vi "usrp_mimo_ofdm_2x1.vi"() -> ()   [LabVIEW 2014]
uses:
  <instrlib>/niUSRP/niUSRP Timestamp.ctl
  <vilib>/addons/Modulation/Analog/controls/Complex Data Waveform.ctl
  <vilib>/addons/Modulation/Digital/General/MT Generate Bits (Galois, PN Order).vi
  <vilib>/addons/Modulation/Digital/Support/Common/Validators/mod_Generate Bits Validate.vi
  <vilib>/addons/Modulation/Analog/support/mod_Set Error Source.vi
  <instrlib>/niUSRP/niUSRP Configure Time Start Trigger.vi
  <vilib>/addons/Modulation/Digital/General/MT Generate QAM System Parameters(M).vi
  <vilib>/addons/Modulation/Digital/Support/Common/Validators/mod_Generate Filter Coefficients Validate.vi
  <vilib>/addons/Modulation/Digital/General/subVIs/mod_Generate Filter Coefficients.vi
  <vilib>/addons/Modulation/Digital/General/subVIs/mod_Generate Bits PN Sequence.vi
  <vilib>/addons/Modulation/Digital/General/MT Map Bits to QAM Symbols.vi
  <vilib>/addons/Modulation/Digital/General/MT Apply Pulse Shaping Filter (Generic).vi
  <instrlib>/niUSRP/niUSRP Write Tx Data (2D CDB).vi
  <instrlib>/niUSRP/niUSRP Fetch Rx Data (2D CDB).vi
  <vilib>/addons/Modulation/Digital/General/MT Apply Matched Filter (Generic).vi
  <vilib>/addons/Modulation/Digital/General/MT Align to Ideal Symbols (Generic).vi
  <vilib>/measure/maspectr.llb/FFT Power Spectrum and PSD for 1 Chan (CDB).vi
  <vilib>/addons/Modulation/Digital/General/MT Map QAM Symbols to Bits.vi
  <vilib>/addons/Modulation/niDMT.lvlib
  <vilib>/measure/NI_MAPro.lvlib
  <vilib>/addons/Modulation/niAMT.lvlib
panel:
  out "Waveform Chart":i16(graph)
  out "size(s) 2":i32
  out "size(s) 3":i32[](array[numeric])
  out "sum":i16
  out "size(s)":i32
  out "x = 0?":bool
  out "input bits stream":i8[](array[numeric]) caption="input bit stream"
  out "output bit stream":i8[](array[numeric])
  in  "CP length":u32=32 caption="CP Size"
  in  "Message Carrier":u32=128
  in  "FFT Size":u32=256
  in  "RXa:Timebase Clock Source":string(combo)="Internal"
  in  "RXa:Reference Frequency Source":string(combo)="Internal"
  in  "TXa:Timebase Clock Source":string(combo)="Internal"
  in  "TXa:Reference Frequency Source":string(combo)="Internal"
  out "OFF":bool=TRUE
  out "RX error":bool
  out "TX error":bool
  out "ERROR":bool
  out "Decoded Constellation Map":cdb[](graph)
  in  "TX timeout":dbl=10.0
  out "error IO":errorcluster
  in  "stop":bool
  out "Transmitted Constellation Map":cluster{dbl[], dbl[]}[](graph)
  out "PSD of Received Signal":cluster{"f0":dbl, "df":dbl, "magnitude":dbl[]}[](graph)
  out "USRP timestamp":T1={"whole seconds"=11, "fractional seconds"=0.9000012199999999}
  in  "number of samples":i64=100000
  in  "M-QAM (16)":i32=16
  in  "total bits (128)":i32=512 caption="total bits (512)"
  in  "filter length (symbols)":i32=8
  in  "filter parameter":dbl=0.5 format="%.2f"
  in  "samples per symbol (16)":i32=4
  in  "pulse shaping filter (none)":T2(ring)=enum."Raised Cosine"
  in  "RXb:Timebase Clock Source":string(combo)="Mimo"
  in  "RXb:Reference Frequency Source":string(combo)="Mimo"
  in  "TXb:Timebase Clock Source":string(combo)="Mimo"
  in  "TXb:Reference Frequency Source":string(combo)="Mimo"
  in  "RXb Active Antenna":string="RX2"
  in  "TXb Active Antenna":string="TX1"
  in  "RXb Gain":dbl
  in  "TXb Gain":dbl
  in  "RXa Active Antenna":string="RX2"
  in  "RXa Gain":dbl
  in  "TXa Active Antenna":string="TX1"
  in  "TXa Gain":dbl
  in  "Carrier Frequency":dbl=1200000000.0 format="%#_6p"
  in  "IQ Rate":dbl=1000000.0 format="%#_6p"
  in  "TX device names":refnum<k15>="192.168.10.2;192.168.10.5"
  in  "start trigger time":T1={"whole seconds"=4, "fractional seconds"=0.1}
  in  "RX device names":refnum<k15>="192.168.10.2;192.168.10.5"
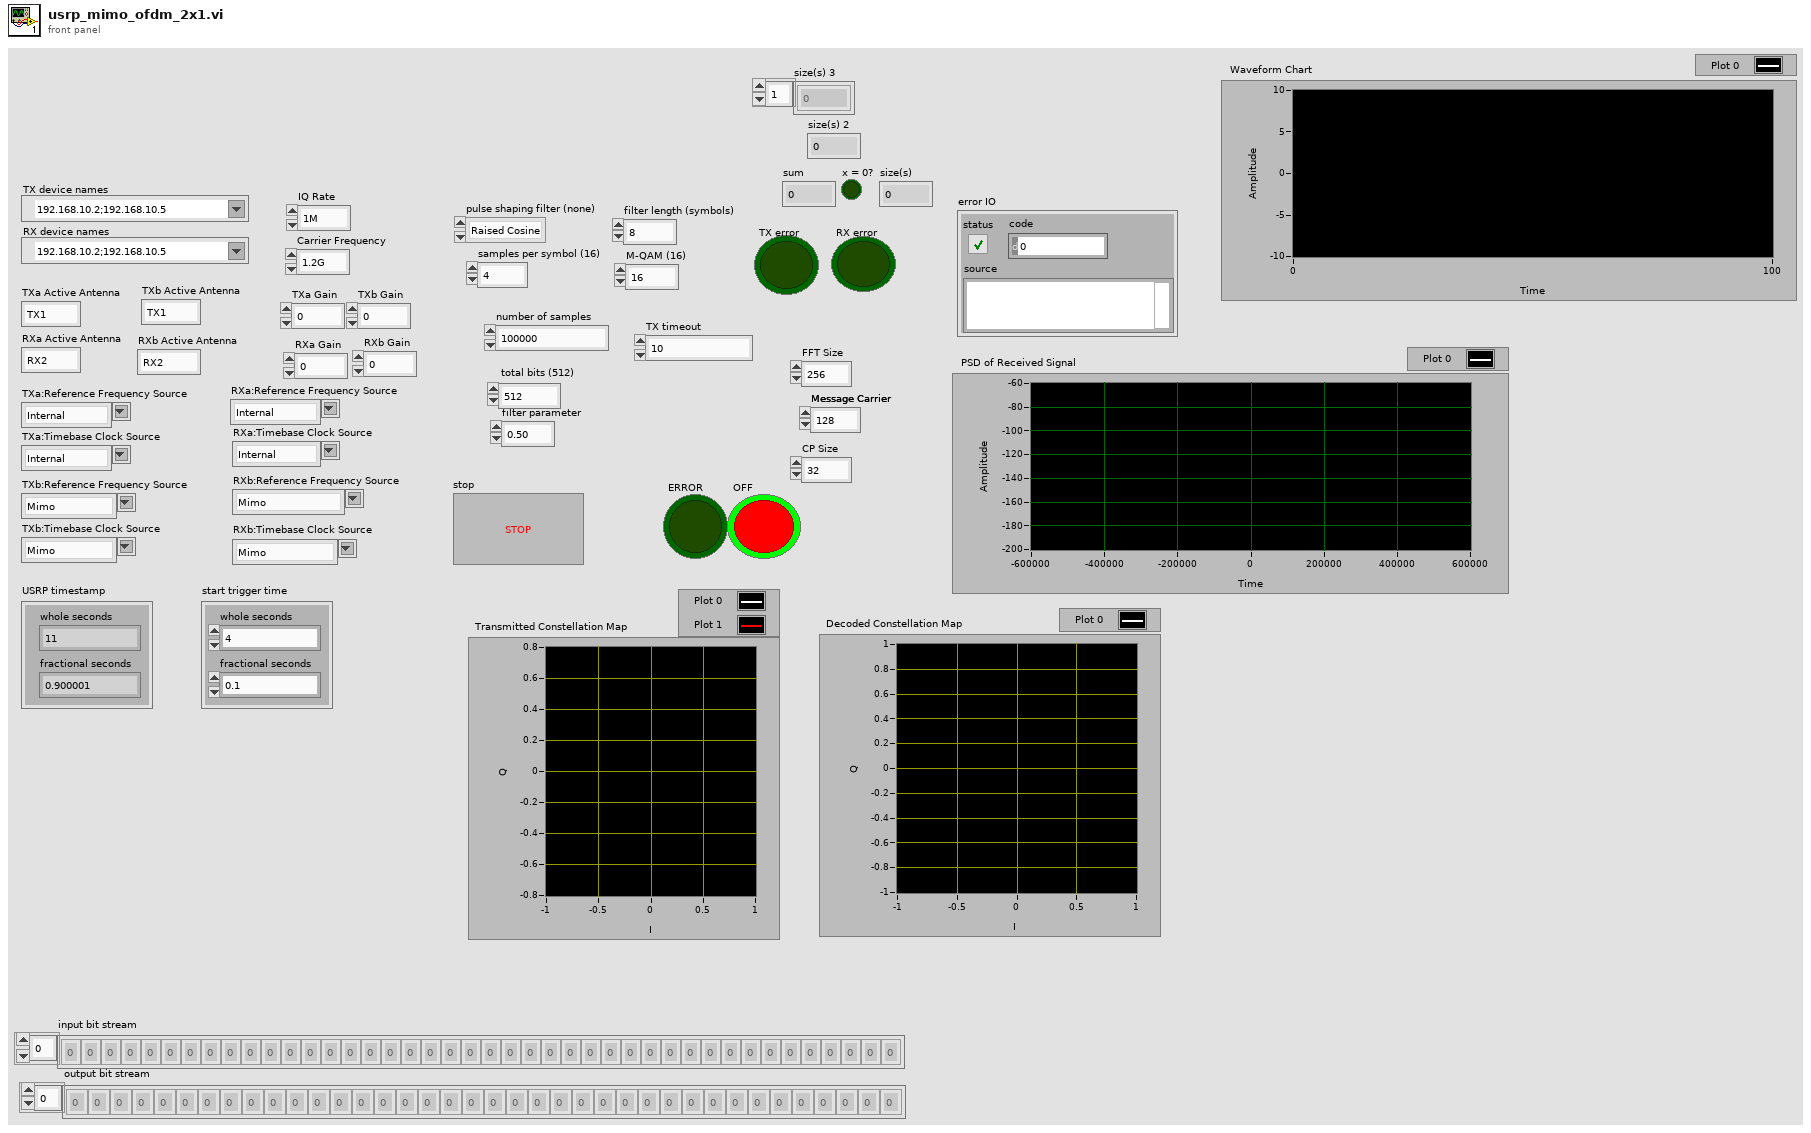
[diagram p1: front panel]
types:
  T1 = typedef "niUSRP Timestamp.ctl" = cluster{"whole seconds":u64, "fractional seconds":dbl}
  T2 = enum16{"none", "Raised Cosine", "Root Raised Cos", "Gaussian"}
  T3 = enum16{"FSK", "PSK", "QAM", "MSK", "PAM", "ASK", "CPM"}
  T4 = cluster{"samples per symbol (16)":i32, "symbol map":cdb[]}
  T5 = typedef "niAMT.lvlib/Complex Data Waveform.ctl" = cluster{"t0":dbl, "dt":dbl, "Y":cdb[]}
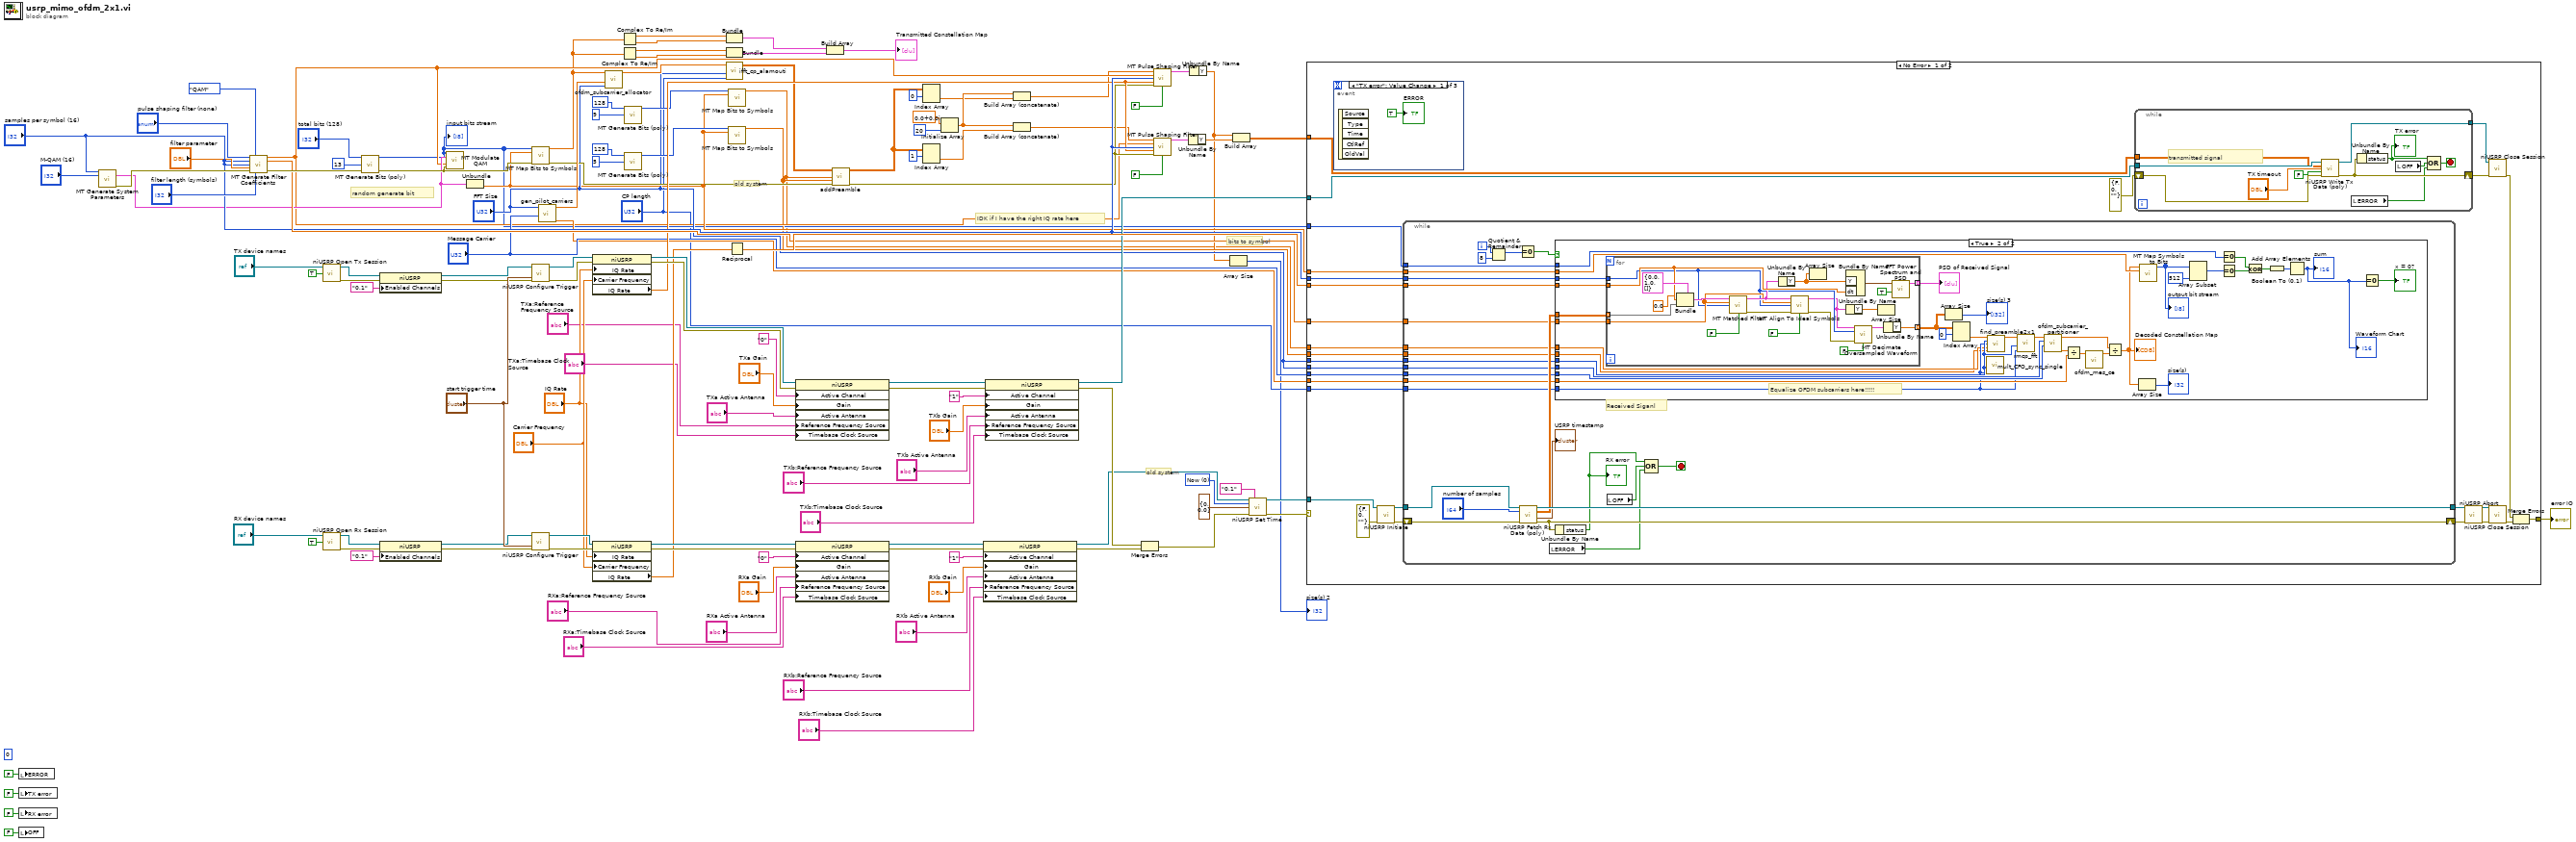
[diagram p0: block diagram]
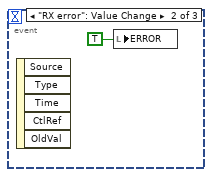
[diagram p2: hidden frame]
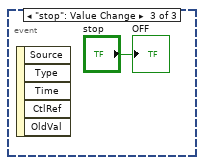
[diagram p3: hidden frame]
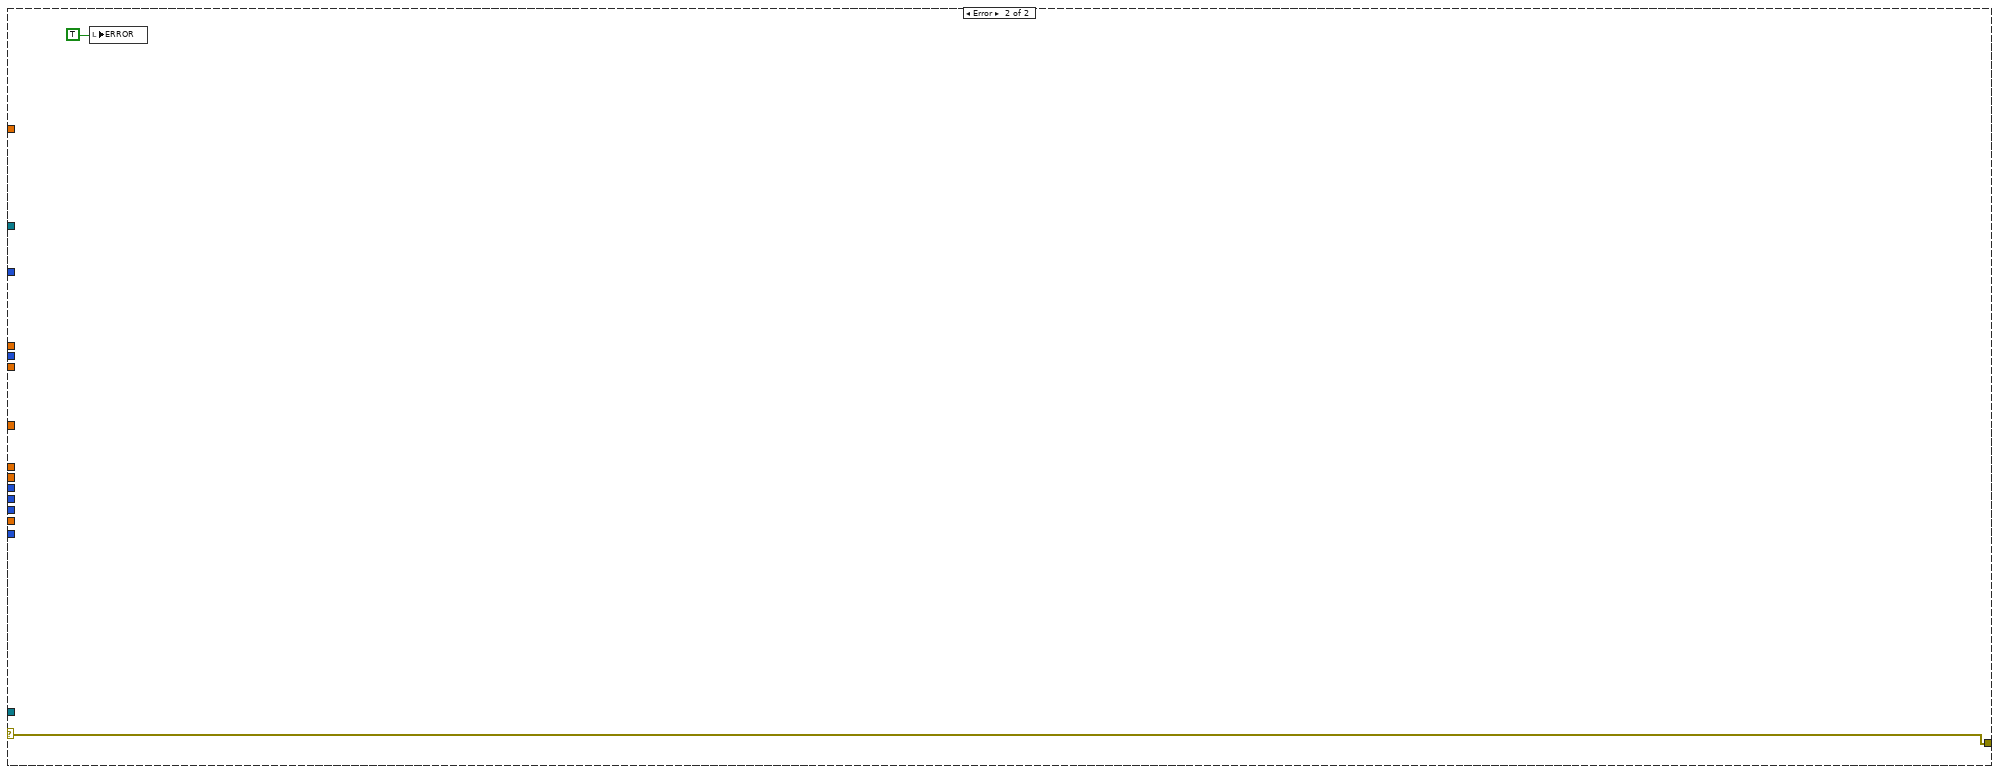
[diagram p5: hidden frame]
diagram:
  (unwired) 0 ("index")
  w85 = 0 items=["Now", "Next Timebase Edge"] ("apply timestamp")
  # "IDK if I have the right IQ rate here"
  # "bits to symbol"
  # "old system"
  # "old system"
  # "random generate bit"
  n1 = local write "ERROR"(FALSE) -> ()
  n2 = local write "TX error"(FALSE) -> ()
  n3 = local write "RX error"(FALSE) -> ()
  n4 = local write "OFF"(FALSE) -> ()
  n5 = call-poly <vilib>:"MT Generate System Parameters.vi"("samples per symbol (16)"="samples per symbol (16)", "M-QAM (16)"="M-QAM (16)") -> ("QAM system parameters"=w27:T4, "error out"=w75:errorcluster)  [unwired: 11 in, 1 out]
  n6 = call <vilib>:"MT Generate Filter Coefficients.vi"("pulse shaping filter (none)"="pulse shaping filter (none)", "modulation type"=T3."QAM", "pulse shaping samples per symbol (16)"="samples per symbol (16)", "matched samples per symbol (16)"="samples per symbol (16)", "filter parameter"="filter parameter", "error in (no error)"=w75, "filter length (symbols)"="filter length (symbols)") -> ("pulse shaping filter coefficients"=w18:dbl[], "matched filter coefficients"=w53:dbl[], "error out"=w74:errorcluster)  [unwired: 6 in]
  n7 = call <instrlib>:"niUSRP Open Tx Session.vi"("device names"="TX device names", "reset"=TRUE) -> ("session handle out"=w58:refnum<k15>, "error out"=w57:errorcluster)  [unwired: 12 in]
  n8 = call <instrlib>:"niUSRP Open Rx Session.vi"("device names"="RX device names", "reset"=TRUE) -> ("session handle out"=w60:refnum<k15>, "error out"=w59:errorcluster)  [unwired: 12 in]
  n9 = call-poly <vilib>:"MT Generate Bits (poly).vi"("total bits (128)"="total bits (128)", "PN sequence order (9)"=13, "error in (no error)"=w74) -> ("output bit stream"=w15:i8[], "error out"=w44:errorcluster)  [unwired: 10 in, 1 out]
  "input bits stream" <- w15
  n10 = property class="niUSRP"(reference=w58, error in=w57, "Enabled Channels"="0,1" ("Configuration:Enabled Channels")) -> (reference out=w119:refnum<k15>, error out=w118:errorcluster)
  n11 = property class="niUSRP"(reference=w60, error in=w59, "Enabled Channels"="0,1" ("Configuration:Enabled Channels")) -> (reference out=w117:refnum<k15>, error out=w116:errorcluster)
  n12 = call <vilib>:"MT Modulate QAM.vi"("input bit stream"=w15, "QAM system parameters"=w27, "pulse shaping filter coefficients"=w18, "error in (no error)"=w44) -> ()  [unwired: 9 in, 3 out]
  n13 = Unbundle(w27) -> ("symbol map"=w21:cdb[])  [unwired: 1 out]
  n14 = call-poly <instrlib>:"niUSRP Configure Trigger.vi"("session handle"=w119, "start trigger time"="start trigger time", "error in (no error)"=w118) -> ("session handle out"=w111:refnum<k15>, "error out"=w110:errorcluster)  [unwired: 11 in]
  n15 = call-poly <instrlib>:"niUSRP Configure Trigger.vi"("session handle"=w117, "start trigger time"="start trigger time", "error in (no error)"=w116) -> ("session handle out"=w115:refnum<k15>, "error out"=w114:errorcluster)  [unwired: 11 in]
  n16 = call-poly <vilib>:"MT Map Bits to Symbols.vi"("input bit stream"=w15, "symbol map"=w21, "error in (no error)"=w44) -> ("symbols"=w16:cdb[], "error out"=w31:errorcluster)  [unwired: 11 in]
  n17 = call "gen_pilot_carriers.vi"("message carrier"="Message Carrier", "FFT size"="FFT Size") -> ("RX pilot carriers"=w22:cdb[], "TX pilot carriers"=w43:cdb[])  [unwired: 8 in]
  n18 = property class="niUSRP"(reference=w111, error in=w110, "IQ Rate"="IQ Rate", "Carrier Frequency"="Carrier Frequency") -> (reference out=w107:refnum<k15>, error out=w106:errorcluster, "IQ Rate"=w38:dbl)
  n19 = property class="niUSRP"(reference=w115, error in=w114, "IQ Rate"="IQ Rate", "Carrier Frequency"="Carrier Frequency") -> (reference out=w113:refnum<k15>, error out=w112:errorcluster, "IQ Rate"=w70:dbl)
  n20 = call "ofdm_subcarrier_allocator.vi"("fft size"="FFT Size", "pilot symbol"=w43, "message symbol"=w16) -> ("OFDM symbol"=w42:cdb[])  [unwired: 8 in]
  n21 = Complex To Re/Im(x + iy=w16) -> (x=w68:dbl[], y=w67:dbl[])
  n22 = Complex To Re/Im(x + iy=w16) -> (x=w66:dbl[], y=w65:dbl[])
  n23 = call-poly <vilib>:"MT Generate Bits (poly).vi"("total bits (128)"=128, "PN sequence order (9)"=9) -> ("output bit stream"=w24:i8[])  [unwired: 11 in, 2 out]
  n24 = call-poly <vilib>:"MT Generate Bits (poly).vi"("total bits (128)"=128, "PN sequence order (9)"=5) -> ("output bit stream"=w26:i8[])  [unwired: 11 in, 2 out]
  n25 = Bundle(w68, w67) -> (w63:cluster{dbl[], dbl[]})  [unwired: 1 in]
  n26 = Bundle(w66, w65) -> (w64:cluster{dbl[], dbl[]})  [unwired: 1 in]
  n27 = call "ifft_cp_alamouti.vi"("CP Length"="CP length", "FFT Size"="FFT Size", "Modulated Stream"=w42) -> ("Baseband Streams"=w33:cdb[][])  [unwired: 8 in]
  n28 = call-poly <vilib>:"MT Map Bits to Symbols.vi"("input bit stream"=w24, "symbol map"=w21) -> ("symbols"=w1:cdb[])  [unwired: 12 in, 1 out]
  n29 = call-poly <vilib>:"MT Map Bits to Symbols.vi"("input bit stream"=w26, "symbol map"=w21) -> ("symbols"=w17:cdb[])  [unwired: 12 in, 1 out]
  n30 = Reciprocal(x=w70) -> (1/x=w69:dbl)
  n31 = property class="niUSRP"(reference=w107, error in=w106, "Active Channel"="0", "Gain"="TXa Gain", "Active Antenna"="TXa Active Antenna", "Reference Frequency Source"="TXa:Reference Frequency Source", "Timebase Clock Source"="TXa:Timebase Clock Source") -> (reference out=w97:refnum<k15>, error out=w96:errorcluster)
  n32 = property class="niUSRP"(reference=w113, error in=w112, "Active Channel"="0", "Gain"="RXa Gain", "Active Antenna"="RXa Active Antenna", "Reference Frequency Source"="RXa:Reference Frequency Source", "Timebase Clock Source"="RXa:Timebase Clock Source") -> (reference out=w99:refnum<k15>, error out=w98:errorcluster)
  n33 = Build Array(w63, w64) -> (→"Transmitted Constellation Map":cluster{dbl[], dbl[]}[])
  n34 = call "addPreamble.vi"("Input Symbol Stream"=w33, "Training Sequence"=w1, "Training Sequence 2"=w17, "error in (no error)"=w31) -> ("Output Transmit \nPackets"=w32:cdb[][], "error out"=w30:errorcluster)  [unwired: 10 in]
  n35 = Index Array(array=w32, index (row)=0) -> (element=w2:cdb[])  [unwired: 1 in]
  n36 = Index Array(array=w32, index (row)=1) -> (element=w3:cdb[])  [unwired: 1 in]
  n37 = Initialize Array(cdb 0.0+0.0i ("element"), 20 ("dimension size")) -> (w4:cdb[])
  n38 = property class="niUSRP"(reference=w99, error in=w98, "Active Channel"="1", "Gain"="RXb Gain", "Active Antenna"="RXb Active Antenna", "Reference Frequency Source"="RXb:Reference Frequency Source", "Timebase Clock Source"="RXb:Timebase Clock Source") -> (reference out=w55:refnum<k15>, error out=w83:errorcluster)
  n39 = property class="niUSRP"(reference=w97, error in=w96, "Active Channel"="1", "Gain"="TXb Gain", "Active Antenna"="TXb Active Antenna", "Reference Frequency Source"="TXb:Reference Frequency Source", "Timebase Clock Source"="TXb:Timebase Clock Source") -> (reference out=w56:refnum<k15>, error out=w82:errorcluster)
  n40 = Build Array (concatenate)(w4, w2) -> (w6:cdb[])
  n41 = Build Array (concatenate)(w4, w3) -> (w5:cdb[])
  n42 = Merge Errors(w82, w83) -> (w81:errorcluster)
  n43 = call-poly <vilib>:"MT Pulse Shaping Filter.vi"("symbols"=w6, "pulse shaping filter coefficients"=w18, "samples per symbol (16)"="samples per symbol (16)", "symbol rate (Hz)"=w38, "error in (no error)"=w30, "reset? (T)"=FALSE) -> ("output complex waveform"=w36:T5)  [unwired: 8 in, 1 out]
  n44 = call-poly <vilib>:"MT Pulse Shaping Filter.vi"("symbols"=w5, "pulse shaping filter coefficients"=w18, "samples per symbol (16)"="samples per symbol (16)", "symbol rate (Hz)"=w38, "error in (no error)"=w30, "reset? (T)"=FALSE) -> ("output complex waveform"=w35:T5)  [unwired: 8 in, 1 out]
  n45 = Unbundle By Name(w35) -> ("Y"=w34:cdb[])
  n46 = Unbundle By Name(w36) -> ("Y"=w10:cdb[])
  n47 = Array Size(array=w10) -> (size(s)=→"size(s) 2":i32)
  n48 = Build Array(w10, w34) -> (w13:cdb[][])
  n49 = call <instrlib>:"niUSRP Set Time.vi"("session handle"=w55, "channel list"="0,1" ("Configuration:Enabled Channels"), "apply timestamp"=w85, "timestamp"=T1 {"whole seconds"=0, "fractional seconds"=0.0}, "error in (no error)"=w81) -> ("session handle out"=w54:refnum<k15>, "error out"=w80:errorcluster)  [unwired: 9 in]
  n50 = case shown="No Error" w80 {
    selector: w80 -> [_ w253]
    tunnel: w54 -> [w140 _]
    tunnel: w56 -> [w153 _]
    tunnel: w13 -> [w154 _]
    tunnel: w69 -> [w144 _]
    tunnel: [w141 w253] -> w62
    tunnel: w53 -> [w137 _]
    tunnel: "samples per symbol (16)" -> [w136 _]
    tunnel: "FFT Size" -> [w135 _]
    tunnel: "Message Carrier" -> [w134 _]
    tunnel: w1 -> [w133 _]
    tunnel: w17 -> [w132 _]
    tunnel: "FFT Size" -> [w131 _]
    tunnel: "CP length" -> [w130 _]
    tunnel: w22 -> [w129 _]
    tunnel: w21 -> [w128 _]
    tunnel: w15 -> [w127 _]
    frame No Error {
      n51 = event shown="[0] \"TX error\": Value Change" {
        selector: _ -> [_ _ _]
        dyn-events: _ -> [_ _ _]
        timeout: _ -> [_ _ _]
        event "TX error": Value Change {
          n52 = event-data() -> ()  [unwired: 1 in, 5 out]
          "ERROR" <- TRUE
        }
        event "RX error": Value Change {
          n53 = event-data() -> ()  [unwired: 1 in, 5 out]
          n54 = local write "ERROR"(TRUE) -> ()
        }
        event "stop": Value Change {
          n55 = event-data() -> ()  [unwired: 1 in, 5 out]
          "OFF" <- "stop"
        }
      }
      n56 = call <instrlib>:"niUSRP Initiate.vi"("session handle"=w140, "error in (no error)"=errorcluster {"status"=FALSE, "code"=0, "source"=""}) -> ("session handle out"=w152:refnum<k15>, "error out"=w151:errorcluster)  [unwired: 12 in]
      n57 = while {
        tunnel: w152 -> [w183]
        shift-right: [w177] -> w150
        shift-left: w151 -> [w182]
        tunnel: [w181] -> w149
        tunnel: w144 -> [w178]
        tunnel: w137 -> [w174]
        tunnel: w136 -> [w173]
        tunnel: w135 -> [w170]
        tunnel: w134 -> [w169]
        tunnel: w133 -> [w168]
        tunnel: w132 -> [w167]
        tunnel: w131 -> [w166]
        tunnel: w130 -> [w165]
        tunnel: w129 -> [w164]
        tunnel: w128 -> [w163]
        tunnel: w127 -> [w162]
        i -> [w161]
        stop <- w175 stop-if-true
        # "Received Siganl"
        n58 = Quotient & Remainder(x=w161, y=8) -> (x-y*floor(x/y)=w159:i32)  [unwired: 1 out]
        n59 = Equal To 0?(x=w159) -> (x = 0?=w158:bool)
        n60 = call-poly <instrlib>:"niUSRP Fetch Rx Data (poly).vi"("session handle"=w183, "number of samples"="number of samples", "error in (no error)"=w182) -> ("session handle out"=w181:refnum<k15>, "data"=w179:cdb[][], "timestamp"=→"USRP timestamp":T1, "error out"=w177:errorcluster)  [unwired: 9 in]
        n61 = local read "ERROR"() -> (w172:bool)
        n62 = case shown="True" w158 {
          tunnel: w179 -> [_ w217]
          tunnel: w178 -> [_ w219]
          tunnel: w174 -> [_ w216]
          tunnel: w173 -> [_ w215]
          tunnel: w170 -> [_ w214]
          tunnel: w169 -> [_ w213]
          tunnel: w168 -> [_ w188]
          tunnel: w167 -> [_ w187]
          tunnel: w166 -> [_ w190]
          tunnel: w165 -> [_ w189]
          tunnel: w164 -> [_ w212]
          tunnel: w163 -> [_ w211]
          tunnel: w162 -> [_ w200]
          frame False {
          }
          frame True {
            # "Equalize OFDM subcarriers here!!!!!"
            n63 = for {
              tunnel: w219 -> [w236]
              tunnel: [w238] -> w218 mode=indexing
              tunnel: w217 -> [w235] mode=indexing
              tunnel: w216 -> [w231]
              tunnel: w215 -> [w228]
              tunnel: [w220] -> w193 mode=indexing
              n64 = Bundle(cluster=T5 {"t0"=0.0, "dt"=1.0, "Y"=[]} ("input complex waveform"), "t0"=0.0, "dt"=w236, "Y"=w235) -> (w233:T5)
              n65 = call-poly <vilib>:"MT Matched Filter.vi"("input complex waveform"=w233, "matched filter coefficients"=w231, "samples per symbol (16)"=w228, "reset? (T)"=FALSE) -> ("output complex waveform"=w232:T5, "error out"=w230:errorcluster)  [unwired: 10 in]
              n66 = Unbundle By Name(w232) -> ("Y"=w223:cdb[])
              n67 = call-poly <vilib>:"MT Align To Ideal Symbols.vi"("input complex waveform"=w232, "matched filter coefficients"=w231, "samples per symbol (16)"=w228, "error in (no error)"=w230, "reset? (T)"=FALSE) -> ("output complex waveform"=w222:T5, "error out"=w229:errorcluster)  [unwired: 8 in, 1 out]
              n68 = Array Size(array=w223) -> ()  [unwired: 1 out]
              n69 = Bundle By Name("Y"=w223, "dt"=w236) -> (w240:waveform(cdb))  [unwired: 1 in]
              n70 = Unbundle By Name(w222) -> ("Y"=w221:cdb[])
              n71 = call <vilib>:"MT Decimate Oversampled Waveform.vi"("input complex waveform"=w222, "decimation factor"=w228, "error in (no error)"=w229, "reset? (T)"=FALSE) -> ("output complex waveform"=w227:T5)  [unwired: 10 in, 1 out]
              n72 = Array Size(array=w221) -> ()  [unwired: 1 out]
              n73 = Unbundle By Name(w227) -> ("Y"=w220:cdb[])
              n74 = call-poly <vilib>:"FFT Power Spectrum and PSD.vi"("dB On (F)"=TRUE, "time signal"=w240) -> ("Power Spectrum / PSD"=w238:cluster{"f0":dbl, "df":dbl, "magnitude":dbl[]})  [unwired: 6 in, 3 out]
            }
            "PSD of Received Signal" <- w218
            n75 = Array Size(array=w193) -> (size(s)=→"size(s) 3":i32[])
            n76 = Index Array(array=w193, index (row)=0) -> (element=w191:cdb[])  [unwired: 1 in]
            n77 = call "mult_CFO_sync_single.vi"("CP length"=w189, "FFT size"=w190) -> ()  [unwired: 9 in, 1 out]
            n78 = call "find_preamble2x1.vi"("received \ntime symbol"=w191, "FFT Size"=w190, "CP Length"=w189, "1st preamble"=w188, "2nd preamble"=w187) -> ("OFDM Symbol"=w186:cdb[])  [unwired: 10 in]
            n79 = call "rmcp_fft.vi"("CP length"=w189, "fft size"=w190, "time symbol"=w186) -> ("freq output"=w202:cdb[])  [unwired: 8 in]
            n80 = call "ofdm_subcarrier_partitioner.vi"("message carrier"=w213, "FFT size"=w214, "received symbol"=w202) -> ("pilot subcarriers"=w207:cdb[], "message subcarriers"=w204:cdb[])  [unwired: 7 in]
            n81 = Divide(x=w207, y=w212) -> (x/y=w206:cdb[])
            n82 = call "ofdm_mes_ce.vi"("ZF \nchannel \nestimates"=w206) -> ("interpolated\n mes carrier CE"=w205:cdb[])  [unwired: 10 in]
            n83 = Divide(x=w204, y=w205) -> (x/y=w201:cdb[])
            "Decoded Constellation Map" <- w201
            n84 = Array Size(array=w201) -> (size(s)=→"size(s)":i32)
            n85 = call-poly <vilib>:"MT Map Symbols to Bits.vi"("symbols"=w201, "symbol map"=w211) -> ("output bit stream"=w209:i8[])  [unwired: 12 in, 1 out]
            "output bit stream" <- w209
            n86 = Array Subset(array=w209, length=512) -> (w198:i8[])  [unwired: 1 in]
            n87 = Equal To 0?(x=w200) -> (x = 0?=w197:bool[])
            n88 = Equal To 0?(x=w198) -> (x = 0?=w199:bool[])
            n89 = Exclusive Or(1:w199, 2:w197) -> (0:w196:bool[])
            n90 = Boolean To (0,1)(Boolean=w196) -> (0, 1=w195:i16[])
            n91 = Add Array Elements(numeric array=w195) -> (sum=w185:i16)
            "sum" <- w185
            "Waveform Chart" <- w185
            n92 = Equal To 0?(x=w185) -> (x = 0?=→"x = 0?":bool)
          }
        }
        n93 = Unbundle By Name(w177) -> ("status"=w176:bool)
        "RX error" <- w176
        n94 = local read "OFF"() -> (w171:bool)
        n95 = Compound Arithmetic op=OR(w176, w171, w172) -> (w175:bool)
      }
      n96 = while {
        tunnel: w154 -> [w247]
        tunnel: w153 -> [w251]
        tunnel: [w250] -> w146
        shift-right: [w246] -> w145
        shift-left: errorcluster {"status"=FALSE, "code"=0, "source"=""} ("error out") -> [w249]
        stop <- w244 stop-if-true
        # "transmitted signal"
        n97 = call-poly <instrlib>:"niUSRP Write Tx Data (poly).vi"("session handle"=w251, "data"=w247, "timeout"="TX timeout", "end of data?"=FALSE, "error in (no error)"=w249) -> ("session handle out"=w250:refnum<k15>, "error out"=w246:errorcluster)  [unwired: 9 in]
        n98 = local read "ERROR"() -> (w242:bool)
        n99 = Unbundle By Name(w246) -> ("status"=w245:bool)
        "TX error" <- w245
        n100 = local read "OFF"() -> (w241:bool)
        n101 = Compound Arithmetic op=OR(w245, w241, w242) -> (w244:bool)
      }
      n102 = call <instrlib>:"niUSRP Abort.vi"("session handle"=w149, "error in (no error)"=w150) -> ("session handle out"=w148:refnum<k15>, "error out"=w147:errorcluster)  [unwired: 12 in]
      n103 = call <instrlib>:"niUSRP Close Session.vi"("session handle"=w146, "error in (no error)"=w145) -> ("error out"=w142:errorcluster)  [unwired: 13 in]
      n104 = call <instrlib>:"niUSRP Close Session.vi"("session handle"=w148, "error in (no error)"=w147) -> ("error out"=w143:errorcluster)  [unwired: 13 in]
      n105 = Merge Errors(w142, w143) -> (w141:errorcluster)
    }
    frame Error {
      n106 = local write "ERROR"(TRUE) -> ()
    }
  }
  "error IO" <- w62
